vi "Self-Test.vi"(8 "error in (no error)":errorcluster, 11 "VISA resource name":refnum<visa-resource-name>) -> (0 "error out":errorcluster, 1 "Self-Test Result Message":string, 2 "Self-Test Result Code":i32, 3 "VISA resource name out":refnum<visa-resource-name>)   [LabVIEW 2016, in "Agilent 34401.lvlib"]
doc: "Runs the instrument's self test routine and returns the test results."
uses:
  <instrlib>/Agilent 34401/Agilent 34401.lvlib
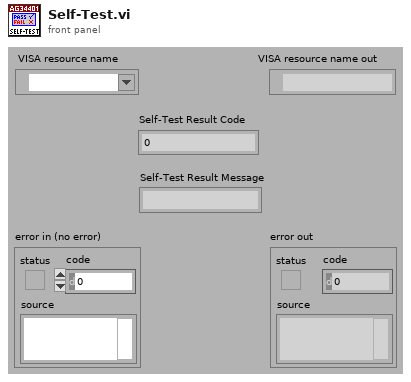
[diagram p1: front panel]
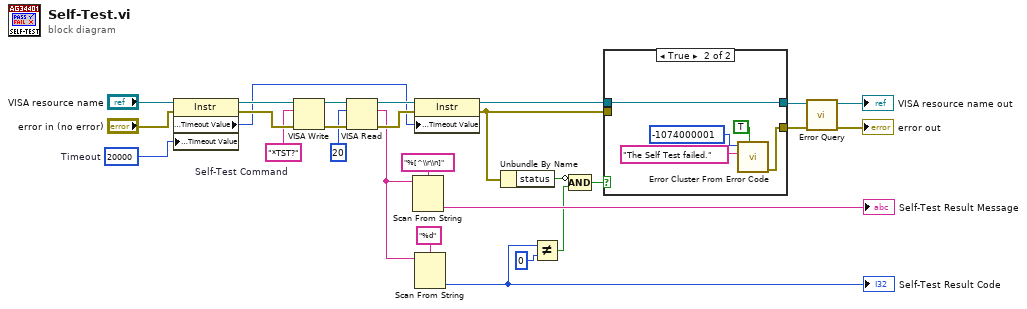
[diagram p0: block diagram]
diagram:
  w14 = u32 20000  # Timeout
  w10 = "*TST?"  # Self-Test Command
  n1 = property on="Property Node" class="Instr"(reference="VISA resource name", error in="error in (no error)", "General Settings:Timeout Value"=w14) -> (reference out=w12:refnum<visa-resource-name>, error out=w13:errorcluster, "General Settings:Timeout Value"=w11:u32)
  n2 = VISA Write(VISA resource name=w12, write buffer=w10, error in (no error)=w13) -> (VISA resource name out=w23:refnum<visa-resource-name>, error out=w22:errorcluster)  [unwired: 1 out]
  n3 = VISA Read(VISA resource name=w23, byte count=u32 20 ("byte count (20)"), error in (no error)=w22) -> (VISA resource name out=w25:refnum<visa-resource-name>, read buffer=w18:string, error out=w24:errorcluster)  [unwired: 1 out]
  n4 = Scan From String(format string="%[^\\r\\n]" ("Format String"), input string=w18) -> (output 1=→"Self-Test Result Message":string)  [unwired: 3 in, 3 out]
  n5 = property on="Property Node" class="Instr"(reference=w25, error in=w24, "General Settings:Timeout Value"=w11) -> (reference out=w2:refnum<visa-resource-name>, error out=w5:errorcluster)
  n6 = Scan From String(format string="%d", input string=w18) -> (output 1=w7:i32)  [unwired: 3 in, 3 out]
  "Self-Test Result Code" <- w7
  n7 = Unbundle By Name(w5) -> ("status"=w8:bool)
  n8 = Not Equal?(x=w7, y=0) -> (x != y?=w9:bool)
  n9 = Compound Arithmetic op=AND(invert w8, w9) -> (w3:bool)
  n10 = case shown="True" w3 {
    tunnel: w5 -> [w29 _]
    tunnel: [w29 w31] -> w4
    tunnel: w2 -> [w28 w30]
    tunnel: [w28 w30] -> w1
    frame False {
    }
    frame True {
      n11 = call <vilib>:"Error Cluster From Error Code.vi"("show call chain? (False)"=TRUE, "error message (\"\")"="The Self Test failed." ("Source (VI Name)"), "error code (0)"=-1074000001 ("Code")) -> ("error out"=w31:errorcluster)  [unwired: 6 in]
    }
  }
  n12 = call <instrlib>:"Error Query.vi"("error in (no error)"=w4, "VISA resource name"=w1) -> ("error out"=→"error out":errorcluster, "VISA resource name out"=→"VISA resource name out":refnum<visa-resource-name>)  [unwired: 6 in, 2 out]
